vi "曲线去两端.vi"(11 "曲线In":cluster{"X":dbl[], "Y":dbl[]}[](array[cluster])) -> (2 "启动曲线":cluster{"X":dbl[], "Y":dbl[]}[](array[cluster]), 3 "曲线Out":cluster{"X":dbl[], "Y":dbl[]}[](array[cluster]))   [LabVIEW 2020]
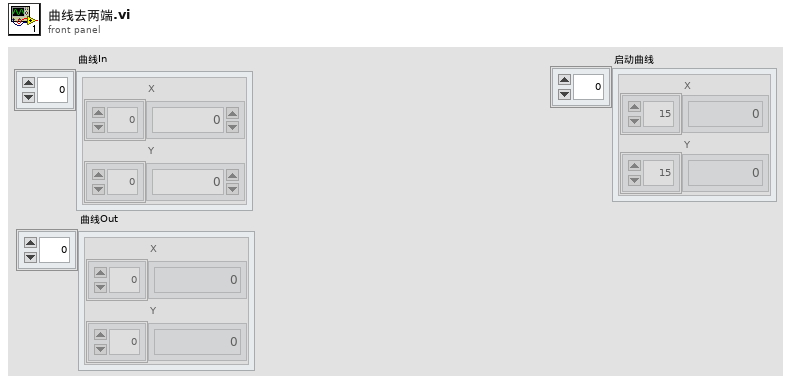
[diagram p1: front panel]
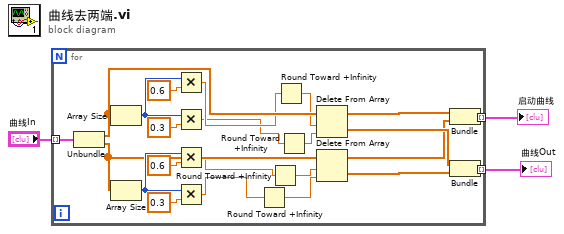
[diagram p0: block diagram]
diagram:
  n1 = for {
    tunnel: "曲线In" -> [w23] mode=indexing
    tunnel: [w15] -> w2 mode=indexing
    tunnel: [w13] -> w1 mode=indexing
    n2 = Unbundle(w23) -> ("X"=w19:dbl[], "Y"=w17:dbl[])
    n3 = Array Size(array=w19) -> (size(s)=w25:i32)
    n4 = Array Size(array=w17) -> (size(s)=w21:i32)
    n5 = Multiply(x=w25, y=0.6) -> (x*y=w11:dbl)
    n6 = Multiply(x=w25, y=0.3) -> (x*y=w5:dbl)
    n7 = Multiply(x=w21, y=0.6) -> (x*y=w7:dbl)
    n8 = Multiply(x=w21, y=0.3) -> (x*y=w9:dbl)
    n9 = Round Toward +Infinity(x=w9) -> (ceil(x): smallest int >= x=w8:dbl)
    n10 = Round Toward +Infinity(x=w7) -> (ceil(x): smallest int >= x=w6:dbl)
    n11 = Round Toward +Infinity(x=w11) -> (ceil(x): smallest int >= x=w10:dbl)
    n12 = Round Toward +Infinity(x=w5) -> (ceil(x): smallest int >= x=w4:dbl)
    n13 = Delete From Array(array=w19, length=w10, index=w4) -> (deleted portion=w18:dbl[], array with subset deleted=w14:dbl[])
    n14 = Delete From Array(array=w17, length=w6, index=w8) -> (deleted portion=w16:dbl[], array with subset deleted=w12:dbl[])
    n15 = Bundle("X"=w14, "Y"=w12) -> (w13:cluster{"X":dbl[], "Y":dbl[]})  [unwired: 1 in]
    n16 = Bundle("X"=w18, "Y"=w16) -> (w15:cluster{"X":dbl[], "Y":dbl[]})  [unwired: 1 in]
  }
  "曲线Out" <- w2
  "启动曲线" <- w1
